vi "dvp Vi Get Trigger Jitter Filter Descr.vi"(6 "pfDefault":dbl, 7 "pfMax":dbl, 9 "pfMin":dbl, 10 "pfStep":dbl, 11 "handle":u32) -> (1 "pfMin out":dbl, 2 "pfStep out":dbl, 3 "function return":u32(ring), 4 "pfDefault out":dbl, 5 "pfMax out":dbl)   [LabVIEW 2018, in "LabViewDVPCamera.lvlib"]
doc: "LabviewDvp2Api dvpStatus dvpViGetTriggerJitterFilterDescr(\n dvpHandle handle, \n double *pfStep,\n double *pfMin,\n double *pfMax,\n double *pfDefault);"
uses:
  LabViewDVPCamera.lvlib
  LabViewDVPCamera/LabViewDVPCamera.dll
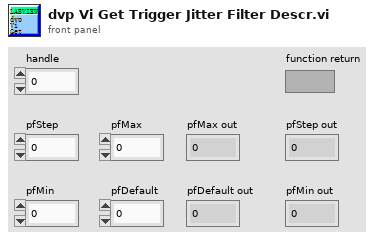
[diagram p1: front panel]
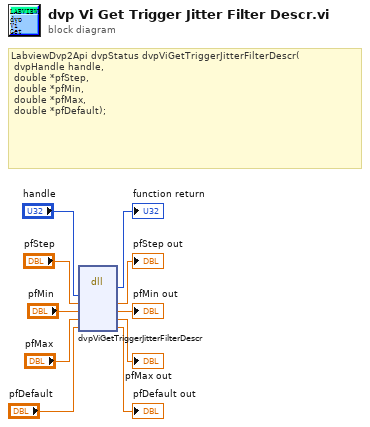
[diagram p0: block diagram]
diagram:
  # "LabviewDvp2Api dvpStatus dvpViGetTriggerJitterFilterDescr(\n\tdvpHandle handle, \n\tdouble *pfStep,\n\tdouble *pfMin,\n\tdouble *pfMax,\n\tdouble *pfDefault);"
  n1 = dll-call lib="C:/Program Files (x86)/DVP2 Labview cn 64/Sample/LabViewDVPCamera/LabViewDVPCamera.*" fn="dvpViGetTriggerJitterFilterDescr"("handle"="handle", "pfStep"="pfStep", "pfMin"="pfMin", "pfMax"="pfMax", "pfDefault"="pfDefault") -> (→"function return":u32, "pfStep"=→"pfStep out":dbl, "pfMin"=→"pfMin out":dbl, "pfMax"=→"pfMax out":dbl, "pfDefault"=→"pfDefault out":dbl)  [unwired: 4 in, 2 out]
